vi "数字量输出配置.vi"() -> ()   [LabVIEW 2010] (continued)
              n515 = local write "单选_第67路"(w31) -> ()
              n516 = local write "单选_第68路"(w31) -> ()
              n517 = local write "单选_第69路"(w31) -> ()
              n518 = local write "单选_第70路"(w31) -> ()
              n519 = local write "单选_第72路"(w31) -> ()
              n520 = local write "单选_第73路"(w31) -> ()
              n521 = local write "单选_第74路"(w31) -> ()
              n522 = local write "单选_第75路"(w31) -> ()
              n523 = local write "单选_第76路"(w31) -> ()
              n524 = local write "单选_第77路"(w31) -> ()
              n525 = local write "单选_第78路"(w31) -> ()
              n526 = local write "单选_第80路"(w31) -> ()
            }
            frame 2 {
              w32 = TRUE
              w33 = FALSE ("单选_第41路")
              n527 = local write "单选_第1路"(w32) -> ()
              n528 = local write "单选_第2路"(w32) -> ()
              n529 = local write "单选_第3路"(w33) -> ()
              n530 = local write "单选_第4路"(w33) -> ()
              n531 = local write "单选_第5路"(w33) -> ()
              n532 = local write "单选_第6路"(w33) -> ()
              n533 = local write "单选_第7路"(w33) -> ()
              n534 = local write "单选_第8路"(w33) -> ()
              n535 = local write "单选_第9路"(w33) -> ()
              n536 = local write "单选_第10路"(w33) -> ()
              n537 = local write "单选_第11路"(w33) -> ()
              n538 = local write "单选_第12路"(w33) -> ()
              n539 = local write "单选_第13路"(w33) -> ()
              n540 = local write "单选_第14路"(w33) -> ()
              n541 = local write "单选_第15路"(w33) -> ()
              n542 = local write "单选_第16路"(w33) -> ()
              n543 = local write "单选_第17路"(w33) -> ()
              n544 = local write "单选_第18路"(w33) -> ()
              n545 = local write "单选_第19路"(w33) -> ()
              n546 = local write "单选_第20路"(w33) -> ()
              n547 = local write "单选_第21路"(w33) -> ()
              n548 = local write "单选_第22路"(w33) -> ()
              n549 = local write "单选_第23路"(w33) -> ()
              n550 = local write "单选_第24路"(w33) -> ()
              n551 = local write "单选_第25路"(w33) -> ()
              n552 = local write "单选_第26路"(w33) -> ()
              n553 = local write "单选_第27路"(w33) -> ()
              n554 = local write "单选_第28路"(w33) -> ()
              n555 = local write "单选_第29路"(w33) -> ()
              n556 = local write "单选_第30路"(w33) -> ()
              n557 = local write "单选_第31路"(w33) -> ()
              n558 = local write "单选_第32路"(w33) -> ()
              n559 = local write "单选_第33路"(w33) -> ()
              n560 = local write "单选_第34路"(w33) -> ()
              n561 = local write "单选_第35路"(w33) -> ()
              n562 = local write "单选_第36路"(w33) -> ()
              n563 = local write "单选_第37路"(w33) -> ()
              n564 = local write "单选_第38路"(w33) -> ()
              n565 = local write "单选_第39路"(w33) -> ()
              n566 = local write "单选_第40路"(w33) -> ()
              n567 = local write "单选_第41路"(w33) -> ()
              n568 = local write "单选_第42路"(w33) -> ()
              n569 = local write "单选_第43路"(w33) -> ()
              n570 = local write "单选_第44路"(w33) -> ()
              n571 = local write "单选_第45路"(w33) -> ()
              n572 = local write "单选_第46路"(w33) -> ()
              n573 = local write "单选_第47路"(w33) -> ()
              n574 = local write "单选_第48路"(w33) -> ()
              n575 = local write "单选_第49路"(w33) -> ()
              n576 = local write "单选_第50路"(w33) -> ()
              n577 = local write "单选_第51路"(w33) -> ()
              n578 = local write "单选_第52路"(w33) -> ()
              n579 = local write "单选_第53路"(w33) -> ()
              n580 = local write "单选_第54路"(w33) -> ()
              n581 = local write "单选_第55路"(w33) -> ()
              n582 = local write "单选_第56路"(w33) -> ()
              n583 = local write "单选_第57路"(w33) -> ()
              n584 = local write "单选_第58路"(w33) -> ()
              n585 = local write "单选_第59路"(w33) -> ()
              n586 = local write "单选_第60路"(w33) -> ()
              n587 = local write "单选_第61路"(w33) -> ()
              n588 = local write "单选_第62路"(w33) -> ()
              n589 = local write "单选_第63路"(w33) -> ()
              n590 = local write "单选_第64路"(w33) -> ()
              n591 = local write "单选_第71路"(w33) -> ()
              n592 = local write "单选_第79路"(w33) -> ()
              n593 = local write "单选_第65路"(w33) -> ()
              n594 = local write "单选_第66路"(w33) -> ()
              n595 = local write "单选_第67路"(w33) -> ()
              n596 = local write "单选_第68路"(w33) -> ()
              n597 = local write "单选_第69路"(w33) -> ()
              n598 = local write "单选_第70路"(w33) -> ()
              n599 = local write "单选_第72路"(w33) -> ()
              n600 = local write "单选_第73路"(w33) -> ()
              n601 = local write "单选_第74路"(w33) -> ()
              n602 = local write "单选_第75路"(w33) -> ()
              n603 = local write "单选_第76路"(w33) -> ()
              n604 = local write "单选_第77路"(w33) -> ()
              n605 = local write "单选_第78路"(w33) -> ()
              n606 = local write "单选_第80路"(w33) -> ()
            }
            frame 3 {
              w34 = TRUE
              w35 = FALSE ("单选_第41路")
              n607 = local write "单选_第1路"(w34) -> ()
              n608 = local write "单选_第2路"(w34) -> ()
              n609 = local write "单选_第3路"(w34) -> ()
              n610 = local write "单选_第4路"(w35) -> ()
              n611 = local write "单选_第5路"(w35) -> ()
              n612 = local write "单选_第6路"(w35) -> ()
              n613 = local write "单选_第7路"(w35) -> ()
              n614 = local write "单选_第8路"(w35) -> ()
              n615 = local write "单选_第9路"(w35) -> ()
              n616 = local write "单选_第10路"(w35) -> ()
              n617 = local write "单选_第11路"(w35) -> ()
              n618 = local write "单选_第12路"(w35) -> ()
              n619 = local write "单选_第13路"(w35) -> ()
              n620 = local write "单选_第14路"(w35) -> ()
              n621 = local write "单选_第15路"(w35) -> ()
              n622 = local write "单选_第16路"(w35) -> ()
              n623 = local write "单选_第17路"(w35) -> ()
              n624 = local write "单选_第18路"(w35) -> ()
              n625 = local write "单选_第19路"(w35) -> ()
              n626 = local write "单选_第20路"(w35) -> ()
              n627 = local write "单选_第21路"(w35) -> ()
              n628 = local write "单选_第22路"(w35) -> ()
              n629 = local write "单选_第23路"(w35) -> ()
              n630 = local write "单选_第24路"(w35) -> ()
              n631 = local write "单选_第25路"(w35) -> ()
              n632 = local write "单选_第26路"(w35) -> ()
              n633 = local write "单选_第27路"(w35) -> ()
              n634 = local write "单选_第28路"(w35) -> ()
              n635 = local write "单选_第29路"(w35) -> ()
              n636 = local write "单选_第30路"(w35) -> ()
              n637 = local write "单选_第31路"(w35) -> ()
              n638 = local write "单选_第32路"(w35) -> ()
              n639 = local write "单选_第33路"(w35) -> ()
              n640 = local write "单选_第34路"(w35) -> ()
              n641 = local write "单选_第35路"(w35) -> ()
              n642 = local write "单选_第36路"(w35) -> ()
              n643 = local write "单选_第37路"(w35) -> ()
              n644 = local write "单选_第38路"(w35) -> ()
              n645 = local write "单选_第39路"(w35) -> ()
              n646 = local write "单选_第40路"(w35) -> ()
              n647 = local write "单选_第41路"(w35) -> ()
              n648 = local write "单选_第42路"(w35) -> ()
              n649 = local write "单选_第43路"(w35) -> ()
              n650 = local write "单选_第44路"(w35) -> ()
              n651 = local write "单选_第45路"(w35) -> ()
              n652 = local write "单选_第46路"(w35) -> ()
              n653 = local write "单选_第47路"(w35) -> ()
              n654 = local write "单选_第48路"(w35) -> ()
              n655 = local write "单选_第49路"(w35) -> ()
              n656 = local write "单选_第50路"(w35) -> ()
              n657 = local write "单选_第51路"(w35) -> ()
              n658 = local write "单选_第52路"(w35) -> ()
              n659 = local write "单选_第53路"(w35) -> ()
              n660 = local write "单选_第54路"(w35) -> ()
              n661 = local write "单选_第55路"(w35) -> ()
              n662 = local write "单选_第56路"(w35) -> ()
              n663 = local write "单选_第57路"(w35) -> ()
              n664 = local write "单选_第58路"(w35) -> ()
              n665 = local write "单选_第59路"(w35) -> ()
              n666 = local write "单选_第60路"(w35) -> ()
              n667 = local write "单选_第61路"(w35) -> ()
              n668 = local write "单选_第62路"(w35) -> ()
              n669 = local write "单选_第63路"(w35) -> ()
              n670 = local write "单选_第64路"(w35) -> ()
              n671 = local write "单选_第71路"(w35) -> ()
              n672 = local write "单选_第79路"(w35) -> ()
              n673 = local write "单选_第65路"(w35) -> ()
              n674 = local write "单选_第66路"(w35) -> ()
              n675 = local write "单选_第67路"(w35) -> ()
              n676 = local write "单选_第68路"(w35) -> ()
              n677 = local write "单选_第69路"(w35) -> ()
              n678 = local write "单选_第70路"(w35) -> ()
              n679 = local write "单选_第72路"(w35) -> ()
              n680 = local write "单选_第73路"(w35) -> ()
              n681 = local write "单选_第74路"(w35) -> ()
              n682 = local write "单选_第75路"(w35) -> ()
              n683 = local write "单选_第76路"(w35) -> ()
              n684 = local write "单选_第77路"(w35) -> ()
              n685 = local write "单选_第78路"(w35) -> ()
              n686 = local write "单选_第80路"(w35) -> ()
            }
            frame 4 {
              w36 = TRUE
              w37 = FALSE ("单选_第41路")
              n687 = local write "单选_第1路"(w36) -> ()
              n688 = local write "单选_第2路"(w36) -> ()
              n689 = local write "单选_第3路"(w36) -> ()
              n690 = local write "单选_第4路"(w36) -> ()
              n691 = local write "单选_第5路"(w37) -> ()
              n692 = local write "单选_第6路"(w37) -> ()
              n693 = local write "单选_第7路"(w37) -> ()
              n694 = local write "单选_第8路"(w37) -> ()
              n695 = local write "单选_第9路"(w37) -> ()
              n696 = local write "单选_第10路"(w37) -> ()
              n697 = local write "单选_第11路"(w37) -> ()
              n698 = local write "单选_第12路"(w37) -> ()
              n699 = local write "单选_第13路"(w37) -> ()
              n700 = local write "单选_第14路"(w37) -> ()
              n701 = local write "单选_第15路"(w37) -> ()
              n702 = local write "单选_第16路"(w37) -> ()
              n703 = local write "单选_第17路"(w37) -> ()
              n704 = local write "单选_第18路"(w37) -> ()
              n705 = local write "单选_第19路"(w37) -> ()
              n706 = local write "单选_第20路"(w37) -> ()
              n707 = local write "单选_第21路"(w37) -> ()
              n708 = local write "单选_第22路"(w37) -> ()
              n709 = local write "单选_第23路"(w37) -> ()
              n710 = local write "单选_第24路"(w37) -> ()
              n711 = local write "单选_第25路"(w37) -> ()
              n712 = local write "单选_第26路"(w37) -> ()
              n713 = local write "单选_第27路"(w37) -> ()
              n714 = local write "单选_第28路"(w37) -> ()
              n715 = local write "单选_第29路"(w37) -> ()
              n716 = local write "单选_第30路"(w37) -> ()
              n717 = local write "单选_第31路"(w37) -> ()
              n718 = local write "单选_第32路"(w37) -> ()
              n719 = local write "单选_第33路"(w37) -> ()
              n720 = local write "单选_第34路"(w37) -> ()
              n721 = local write "单选_第35路"(w37) -> ()
              n722 = local write "单选_第36路"(w37) -> ()
              n723 = local write "单选_第37路"(w37) -> ()
              n724 = local write "单选_第38路"(w37) -> ()
              n725 = local write "单选_第39路"(w37) -> ()
              n726 = local write "单选_第40路"(w37) -> ()
              n727 = local write "单选_第41路"(w37) -> ()
              n728 = local write "单选_第42路"(w37) -> ()
              n729 = local write "单选_第43路"(w37) -> ()
              n730 = local write "单选_第44路"(w37) -> ()
              n731 = local write "单选_第45路"(w37) -> ()
              n732 = local write "单选_第46路"(w37) -> ()
              n733 = local write "单选_第47路"(w37) -> ()
              n734 = local write "单选_第48路"(w37) -> ()
              n735 = local write "单选_第49路"(w37) -> ()
              n736 = local write "单选_第50路"(w37) -> ()
              n737 = local write "单选_第51路"(w37) -> ()
              n738 = local write "单选_第52路"(w37) -> ()
              n739 = local write "单选_第53路"(w37) -> ()
              n740 = local write "单选_第54路"(w37) -> ()
              n741 = local write "单选_第55路"(w37) -> ()
              n742 = local write "单选_第56路"(w37) -> ()
              n743 = local write "单选_第57路"(w37) -> ()
              n744 = local write "单选_第58路"(w37) -> ()
              n745 = local write "单选_第59路"(w37) -> ()
              n746 = local write "单选_第60路"(w37) -> ()
              n747 = local write "单选_第61路"(w37) -> ()
              n748 = local write "单选_第62路"(w37) -> ()
              n749 = local write "单选_第63路"(w37) -> ()
              n750 = local write "单选_第64路"(w37) -> ()
              n751 = local write "单选_第71路"(w37) -> ()
              n752 = local write "单选_第79路"(w37) -> ()
              n753 = local write "单选_第65路"(w37) -> ()
              n754 = local write "单选_第66路"(w37) -> ()
              n755 = local write "单选_第67路"(w37) -> ()
              n756 = local write "单选_第68路"(w37) -> ()
              n757 = local write "单选_第69路"(w37) -> ()
              n758 = local write "单选_第70路"(w37) -> ()
              n759 = local write "单选_第72路"(w37) -> ()
              n760 = local write "单选_第73路"(w37) -> ()
              n761 = local write "单选_第74路"(w37) -> ()
              n762 = local write "单选_第75路"(w37) -> ()
              n763 = local write "单选_第76路"(w37) -> ()
              n764 = local write "单选_第77路"(w37) -> ()
              n765 = local write "单选_第78路"(w37) -> ()
              n766 = local write "单选_第80路"(w37) -> ()
            }
            frame 5 {
              w38 = TRUE
              w39 = FALSE ("单选_第41路")
              n767 = local write "单选_第1路"(w38) -> ()
              n768 = local write "单选_第2路"(w38) -> ()
              n769 = local write "单选_第3路"(w38) -> ()
              n770 = local write "单选_第4路"(w38) -> ()
              n771 = local write "单选_第5路"(w38) -> ()
              n772 = local write "单选_第6路"(w39) -> ()
              n773 = local write "单选_第7路"(w39) -> ()
              n774 = local write "单选_第8路"(w39) -> ()
              n775 = local write "单选_第9路"(w39) -> ()
              n776 = local write "单选_第10路"(w39) -> ()
              n777 = local write "单选_第11路"(w39) -> ()
              n778 = local write "单选_第12路"(w39) -> ()
              n779 = local write "单选_第13路"(w39) -> ()
              n780 = local write "单选_第14路"(w39) -> ()
              n781 = local write "单选_第15路"(w39) -> ()
              n782 = local write "单选_第16路"(w39) -> ()
              n783 = local write "单选_第17路"(w39) -> ()
              n784 = local write "单选_第18路"(w39) -> ()
              n785 = local write "单选_第19路"(w39) -> ()
              n786 = local write "单选_第20路"(w39) -> ()
              n787 = local write "单选_第21路"(w39) -> ()
              n788 = local write "单选_第22路"(w39) -> ()
              n789 = local write "单选_第23路"(w39) -> ()
              n790 = local write "单选_第24路"(w39) -> ()
              n791 = local write "单选_第25路"(w39) -> ()
              n792 = local write "单选_第26路"(w39) -> ()
              n793 = local write "单选_第27路"(w39) -> ()
              n794 = local write "单选_第28路"(w39) -> ()
              n795 = local write "单选_第29路"(w39) -> ()
              n796 = local write "单选_第30路"(w39) -> ()
              n797 = local write "单选_第31路"(w39) -> ()
              n798 = local write "单选_第32路"(w39) -> ()
              n799 = local write "单选_第33路"(w39) -> ()
              n800 = local write "单选_第34路"(w39) -> ()
              n801 = local write "单选_第35路"(w39) -> ()
              n802 = local write "单选_第36路"(w39) -> ()
              n803 = local write "单选_第37路"(w39) -> ()
              n804 = local write "单选_第38路"(w39) -> ()
              n805 = local write "单选_第39路"(w39) -> ()
              n806 = local write "单选_第40路"(w39) -> ()
              n807 = local write "单选_第41路"(w39) -> ()
              n808 = local write "单选_第42路"(w39) -> ()
              n809 = local write "单选_第43路"(w39) -> ()
              n810 = local write "单选_第44路"(w39) -> ()
              n811 = local write "单选_第45路"(w39) -> ()
              n812 = local write "单选_第46路"(w39) -> ()
              n813 = local write "单选_第47路"(w39) -> ()
              n814 = local write "单选_第48路"(w39) -> ()
              n815 = local write "单选_第49路"(w39) -> ()
              n816 = local write "单选_第50路"(w39) -> ()
              n817 = local write "单选_第51路"(w39) -> ()
              n818 = local write "单选_第52路"(w39) -> ()
              n819 = local write "单选_第53路"(w39) -> ()
              n820 = local write "单选_第54路"(w39) -> ()
              n821 = local write "单选_第55路"(w39) -> ()
              n822 = local write "单选_第56路"(w39) -> ()
              n823 = local write "单选_第57路"(w39) -> ()
              n824 = local write "单选_第58路"(w39) -> ()
              n825 = local write "单选_第59路"(w39) -> ()
              n826 = local write "单选_第60路"(w39) -> ()
              n827 = local write "单选_第61路"(w39) -> ()
              n828 = local write "单选_第62路"(w39) -> ()
              n829 = local write "单选_第63路"(w39) -> ()
              n830 = local write "单选_第64路"(w39) -> ()
              n831 = local write "单选_第71路"(w39) -> ()
              n832 = local write "单选_第79路"(w39) -> ()
              n833 = local write "单选_第65路"(w39) -> ()
              n834 = local write "单选_第66路"(w39) -> ()
              n835 = local write "单选_第67路"(w39) -> ()
              n836 = local write "单选_第68路"(w39) -> ()
              n837 = local write "单选_第69路"(w39) -> ()
              n838 = local write "单选_第70路"(w39) -> ()
              n839 = local write "单选_第72路"(w39) -> ()
              n840 = local write "单选_第73路"(w39) -> ()
              n841 = local write "单选_第74路"(w39) -> ()
              n842 = local write "单选_第75路"(w39) -> ()
              n843 = local write "单选_第76路"(w39) -> ()
              n844 = local write "单选_第77路"(w39) -> ()
              n845 = local write "单选_第78路"(w39) -> ()
              n846 = local write "单选_第80路"(w39) -> ()
            }
            frame 6 {
              w40 = TRUE
              w41 = FALSE ("单选_第41路")
              n847 = local write "单选_第1路"(w40) -> ()
              n848 = local write "单选_第2路"(w40) -> ()
              n849 = local write "单选_第3路"(w40) -> ()
              n850 = local write "单选_第4路"(w40) -> ()
              n851 = local write "单选_第5路"(w40) -> ()
              n852 = local write "单选_第6路"(w40) -> ()
              n853 = local write "单选_第7路"(w41) -> ()
              n854 = local write "单选_第8路"(w41) -> ()
              n855 = local write "单选_第9路"(w41) -> ()
              n856 = local write "单选_第10路"(w41) -> ()
              n857 = local write "单选_第11路"(w41) -> ()
              n858 = local write "单选_第12路"(w41) -> ()
              n859 = local write "单选_第13路"(w41) -> ()
              n860 = local write "单选_第14路"(w41) -> ()
              n861 = local write "单选_第15路"(w41) -> ()
              n862 = local write "单选_第16路"(w41) -> ()
              n863 = local write "单选_第17路"(w41) -> ()
              n864 = local write "单选_第18路"(w41) -> ()
              n865 = local write "单选_第19路"(w41) -> ()
              n866 = local write "单选_第20路"(w41) -> ()
              n867 = local write "单选_第21路"(w41) -> ()
              n868 = local write "单选_第22路"(w41) -> ()
              n869 = local write "单选_第23路"(w41) -> ()
              n870 = local write "单选_第24路"(w41) -> ()
              n871 = local write "单选_第25路"(w41) -> ()
              n872 = local write "单选_第26路"(w41) -> ()
              n873 = local write "单选_第27路"(w41) -> ()
              n874 = local write "单选_第28路"(w41) -> ()
              n875 = local write "单选_第29路"(w41) -> ()
              n876 = local write "单选_第30路"(w41) -> ()
              n877 = local write "单选_第31路"(w41) -> ()
              n878 = local write "单选_第32路"(w41) -> ()
              n879 = local write "单选_第33路"(w41) -> ()
              n880 = local write "单选_第34路"(w41) -> ()
              n881 = local write "单选_第35路"(w41) -> ()
              n882 = local write "单选_第36路"(w41) -> ()
              n883 = local write "单选_第37路"(w41) -> ()
              n884 = local write "单选_第38路"(w41) -> ()
              n885 = local write "单选_第39路"(w41) -> ()
              n886 = local write "单选_第40路"(w41) -> ()
              n887 = local write "单选_第41路"(w41) -> ()
              n888 = local write "单选_第42路"(w41) -> ()
              n889 = local write "单选_第43路"(w41) -> ()
              n890 = local write "单选_第44路"(w41) -> ()
              n891 = local write "单选_第45路"(w41) -> ()
              n892 = local write "单选_第46路"(w41) -> ()
              n893 = local write "单选_第47路"(w41) -> ()
              n894 = local write "单选_第48路"(w41) -> ()
              n895 = local write "单选_第49路"(w41) -> ()
              n896 = local write "单选_第50路"(w41) -> ()
              n897 = local write "单选_第51路"(w41) -> ()
              n898 = local write "单选_第52路"(w41) -> ()
              n899 = local write "单选_第53路"(w41) -> ()
              n900 = local write "单选_第54路"(w41) -> ()
              n901 = local write "单选_第55路"(w41) -> ()
              n902 = local write "单选_第56路"(w41) -> ()
              n903 = local write "单选_第57路"(w41) -> ()
              n904 = local write "单选_第58路"(w41) -> ()
              n905 = local write "单选_第59路"(w41) -> ()
              n906 = local write "单选_第60路"(w41) -> ()
              n907 = local write "单选_第61路"(w41) -> ()
              n908 = local write "单选_第62路"(w41) -> ()
              n909 = local write "单选_第63路"(w41) -> ()
              n910 = local write "单选_第64路"(w41) -> ()
              n911 = local write "单选_第71路"(w41) -> ()
              n912 = local write "单选_第79路"(w41) -> ()
              n913 = local write "单选_第65路"(w41) -> ()
              n914 = local write "单选_第66路"(w41) -> ()
              n915 = local write "单选_第67路"(w41) -> ()
              n916 = local write "单选_第68路"(w41) -> ()
              n917 = local write "单选_第69路"(w41) -> ()
              n918 = local write "单选_第70路"(w41) -> ()
              n919 = local write "单选_第72路"(w41) -> ()
              n920 = local write "单选_第73路"(w41) -> ()
              n921 = local write "单选_第74路"(w41) -> ()
              n922 = local write "单选_第75路"(w41) -> ()
              n923 = local write "单选_第76路"(w41) -> ()
              n924 = local write "单选_第77路"(w41) -> ()
              n925 = local write "单选_第78路"(w41) -> ()
              n926 = local write "单选_第80路"(w41) -> ()
            }
            frame 7 {
              w42 = TRUE
              w43 = FALSE ("单选_第41路")
              n927 = local write "单选_第1路"(w42) -> ()
              n928 = local write "单选_第2路"(w42) -> ()
              n929 = local write "单选_第3路"(w42) -> ()
              n930 = local write "单选_第4路"(w42) -> ()
              n931 = local write "单选_第5路"(w42) -> ()
              n932 = local write "单选_第6路"(w42) -> ()
              n933 = local write "单选_第7路"(w42) -> ()
              n934 = local write "单选_第8路"(w43) -> ()
              n935 = local write "单选_第9路"(w43) -> ()
              n936 = local write "单选_第10路"(w43) -> ()
              n937 = local write "单选_第11路"(w43) -> ()
              n938 = local write "单选_第12路"(w43) -> ()
              n939 = local write "单选_第13路"(w43) -> ()
              n940 = local write "单选_第14路"(w43) -> ()
              n941 = local write "单选_第15路"(w43) -> ()
              n942 = local write "单选_第16路"(w43) -> ()
              n943 = local write "单选_第17路"(w43) -> ()
              n944 = local write "单选_第18路"(w43) -> ()
              n945 = local write "单选_第19路"(w43) -> ()
              n946 = local write "单选_第20路"(w43) -> ()
              n947 = local write "单选_第21路"(w43) -> ()
              n948 = local write "单选_第22路"(w43) -> ()
              n949 = local write "单选_第23路"(w43) -> ()
              n950 = local write "单选_第24路"(w43) -> ()
              n951 = local write "单选_第25路"(w43) -> ()
              n952 = local write "单选_第26路"(w43) -> ()
              n953 = local write "单选_第27路"(w43) -> ()
              n954 = local write "单选_第28路"(w43) -> ()
              n955 = local write "单选_第29路"(w43) -> ()
              n956 = local write "单选_第30路"(w43) -> ()
              n957 = local write "单选_第31路"(w43) -> ()
              n958 = local write "单选_第32路"(w43) -> ()
              n959 = local write "单选_第33路"(w43) -> ()
              n960 = local write "单选_第34路"(w43) -> ()
              n961 = local write "单选_第35路"(w43) -> ()
              n962 = local write "单选_第36路"(w43) -> ()
              n963 = local write "单选_第37路"(w43) -> ()
              n964 = local write "单选_第38路"(w43) -> ()
              n965 = local write "单选_第39路"(w43) -> ()
              n966 = local write "单选_第40路"(w43) -> ()
              n967 = local write "单选_第41路"(w43) -> ()
              n968 = local write "单选_第42路"(w43) -> ()
              n969 = local write "单选_第43路"(w43) -> ()
              n970 = local write "单选_第44路"(w43) -> ()
              n971 = local write "单选_第45路"(w43) -> ()
              n972 = local write "单选_第46路"(w43) -> ()
              n973 = local write "单选_第47路"(w43) -> ()
              n974 = local write "单选_第48路"(w43) -> ()
              n975 = local write "单选_第49路"(w43) -> ()
              n976 = local write "单选_第50路"(w43) -> ()
              n977 = local write "单选_第51路"(w43) -> ()
              n978 = local write "单选_第52路"(w43) -> ()
              n979 = local write "单选_第53路"(w43) -> ()
              n980 = local write "单选_第54路"(w43) -> ()
              n981 = local write "单选_第55路"(w43) -> ()
              n982 = local write "单选_第56路"(w43) -> ()
              n983 = local write "单选_第57路"(w43) -> ()
              n984 = local write "单选_第58路"(w43) -> ()
              n985 = local write "单选_第59路"(w43) -> ()
              n986 = local write "单选_第60路"(w43) -> ()
              n987 = local write "单选_第61路"(w43) -> ()
              n988 = local write "单选_第62路"(w43) -> ()
              n989 = local write "单选_第63路"(w43) -> ()
              n990 = local write "单选_第64路"(w43) -> ()
              n991 = local write "单选_第71路"(w43) -> ()
              n992 = local write "单选_第79路"(w43) -> ()
              n993 = local write "单选_第65路"(w43) -> ()
              n994 = local write "单选_第66路"(w43) -> ()
              n995 = local write "单选_第67路"(w43) -> ()
              n996 = local write "单选_第68路"(w43) -> ()
              n997 = local write "单选_第69路"(w43) -> ()
              n998 = local write "单选_第70路"(w43) -> ()
              n999 = local write "单选_第72路"(w43) -> ()
              n1000 = local write "单选_第73路"(w43) -> ()
              n1001 = local write "单选_第74路"(w43) -> ()
              n1002 = local write "单选_第75路"(w43) -> ()
              n1003 = local write "单选_第76路"(w43) -> ()
              n1004 = local write "单选_第77路"(w43) -> ()
              n1005 = local write "单选_第78路"(w43) -> ()
              n1006 = local write "单选_第80路"(w43) -> ()
            }
            frame 8 {
              w44 = TRUE
              w45 = FALSE ("单选_第41路")
              n1007 = local write "单选_第1路"(w44) -> ()
              n1008 = local write "单选_第2路"(w44) -> ()
              n1009 = local write "单选_第3路"(w44) -> ()
              n1010 = local write "单选_第4路"(w44) -> ()
              n1011 = local write "单选_第5路"(w44) -> ()
              n1012 = local write "单选_第6路"(w44) -> ()
              n1013 = local write "单选_第7路"(w44) -> ()
              n1014 = local write "单选_第8路"(w44) -> ()
              n1015 = local write "单选_第9路"(w45) -> ()
              n1016 = local write "单选_第10路"(w45) -> ()
              n1017 = local write "单选_第11路"(w45) -> ()
              n1018 = local write "单选_第12路"(w45) -> ()
              n1019 = local write "单选_第13路"(w45) -> ()
              n1020 = local write "单选_第14路"(w45) -> ()
              n1021 = local write "单选_第15路"(w45) -> ()
              n1022 = local write "单选_第16路"(w45) -> ()
              n1023 = local write "单选_第17路"(w45) -> ()
              n1024 = local write "单选_第18路"(w45) -> ()
              n1025 = local write "单选_第19路"(w45) -> ()
              n1026 = local write "单选_第20路"(w45) -> ()
              n1027 = local write "单选_第21路"(w45) -> ()
              n1028 = local write "单选_第22路"(w45) -> ()
              n1029 = local write "单选_第23路"(w45) -> ()
              n1030 = local write "单选_第24路"(w45) -> ()
              n1031 = local write "单选_第25路"(w45) -> ()
              n1032 = local write "单选_第26路"(w45) -> ()
              n1033 = local write "单选_第27路"(w45) -> ()
              n1034 = local write "单选_第28路"(w45) -> ()
              n1035 = local write "单选_第29路"(w45) -> ()
              n1036 = local write "单选_第30路"(w45) -> ()
              n1037 = local write "单选_第31路"(w45) -> ()
              n1038 = local write "单选_第32路"(w45) -> ()
              n1039 = local write "单选_第33路"(w45) -> ()
              n1040 = local write "单选_第34路"(w45) -> ()
              n1041 = local write "单选_第35路"(w45) -> ()
              n1042 = local write "单选_第36路"(w45) -> ()
              n1043 = local write "单选_第37路"(w45) -> ()
              n1044 = local write "单选_第38路"(w45) -> ()
              n1045 = local write "单选_第39路"(w45) -> ()
              n1046 = local write "单选_第40路"(w45) -> ()
              n1047 = local write "单选_第41路"(w45) -> ()
              n1048 = local write "单选_第42路"(w45) -> ()
              n1049 = local write "单选_第43路"(w45) -> ()
              n1050 = local write "单选_第44路"(w45) -> ()
              n1051 = local write "单选_第45路"(w45) -> ()
              n1052 = local write "单选_第46路"(w45) -> ()
              n1053 = local write "单选_第47路"(w45) -> ()
              n1054 = local write "单选_第48路"(w45) -> ()
              n1055 = local write "单选_第49路"(w45) -> ()
              n1056 = local write "单选_第50路"(w45) -> ()
              n1057 = local write "单选_第51路"(w45) -> ()
              n1058 = local write "单选_第52路"(w45) -> ()
              n1059 = local write "单选_第53路"(w45) -> ()
              n1060 = local write "单选_第54路"(w45) -> ()
              n1061 = local write "单选_第55路"(w45) -> ()
              n1062 = local write "单选_第56路"(w45) -> ()
              n1063 = local write "单选_第57路"(w45) -> ()
              n1064 = local write "单选_第58路"(w45) -> ()
              n1065 = local write "单选_第59路"(w45) -> ()
              n1066 = local write "单选_第60路"(w45) -> ()
              n1067 = local write "单选_第61路"(w45) -> ()
              n1068 = local write "单选_第62路"(w45) -> ()
              n1069 = local write "单选_第63路"(w45) -> ()
              n1070 = local write "单选_第64路"(w45) -> ()
              n1071 = local write "单选_第71路"(w45) -> ()
              n1072 = local write "单选_第79路"(w45) -> ()
              n1073 = local write "单选_第65路"(w45) -> ()
              n1074 = local write "单选_第66路"(w45) -> ()
              n1075 = local write "单选_第67路"(w45) -> ()
              n1076 = local write "单选_第68路"(w45) -> ()
              n1077 = local write "单选_第69路"(w45) -> ()
              n1078 = local write "单选_第70路"(w45) -> ()
              n1079 = local write "单选_第72路"(w45) -> ()
              n1080 = local write "单选_第73路"(w45) -> ()
              n1081 = local write "单选_第74路"(w45) -> ()
              n1082 = local write "单选_第75路"(w45) -> ()
              n1083 = local write "单选_第76路"(w45) -> ()
              n1084 = local write "单选_第77路"(w45) -> ()
              n1085 = local write "单选_第78路"(w45) -> ()
              n1086 = local write "单选_第80路"(w45) -> ()
            }
            frame 9 {
              w46 = TRUE
              w47 = FALSE ("单选_第41路")
              n1087 = local write "单选_第1路"(w46) -> ()
              n1088 = local write "单选_第2路"(w46) -> ()
              n1089 = local write "单选_第3路"(w46) -> ()
              n1090 = local write "单选_第4路"(w46) -> ()
              n1091 = local write "单选_第5路"(w46) -> ()
              n1092 = local write "单选_第6路"(w46) -> ()
              n1093 = local write "单选_第7路"(w46) -> ()
              n1094 = local write "单选_第8路"(w46) -> ()
              n1095 = local write "单选_第9路"(w46) -> ()
              n1096 = local write "单选_第10路"(w47) -> ()
              n1097 = local write "单选_第11路"(w47) -> ()
              n1098 = local write "单选_第12路"(w47) -> ()
              n1099 = local write "单选_第13路"(w47) -> ()
              n1100 = local write "单选_第14路"(w47) -> ()
              n1101 = local write "单选_第15路"(w47) -> ()
              n1102 = local write "单选_第16路"(w47) -> ()
              n1103 = local write "单选_第17路"(w47) -> ()
              n1104 = local write "单选_第18路"(w47) -> ()
              n1105 = local write "单选_第19路"(w47) -> ()
              n1106 = local write "单选_第20路"(w47) -> ()
              n1107 = local write "单选_第21路"(w47) -> ()
              n1108 = local write "单选_第22路"(w47) -> ()
              n1109 = local write "单选_第23路"(w47) -> ()
              n1110 = local write "单选_第24路"(w47) -> ()
              n1111 = local write "单选_第25路"(w47) -> ()
              n1112 = local write "单选_第26路"(w47) -> ()
              n1113 = local write "单选_第27路"(w47) -> ()
              n1114 = local write "单选_第28路"(w47) -> ()
              n1115 = local write "单选_第29路"(w47) -> ()
              n1116 = local write "单选_第30路"(w47) -> ()
              n1117 = local write "单选_第31路"(w47) -> ()
              n1118 = local write "单选_第32路"(w47) -> ()
              n1119 = local write "单选_第33路"(w47) -> ()
              n1120 = local write "单选_第34路"(w47) -> ()
              n1121 = local write "单选_第35路"(w47) -> ()
              n1122 = local write "单选_第36路"(w47) -> ()
              n1123 = local write "单选_第37路"(w47) -> ()
              n1124 = local write "单选_第38路"(w47) -> ()
              n1125 = local write "单选_第39路"(w47) -> ()
              n1126 = local write "单选_第40路"(w47) -> ()
              n1127 = local write "单选_第41路"(w47) -> ()
              n1128 = local write "单选_第42路"(w47) -> ()
              n1129 = local write "单选_第43路"(w47) -> ()
              n1130 = local write "单选_第44路"(w47) -> ()
              n1131 = local write "单选_第45路"(w47) -> ()
              n1132 = local write "单选_第46路"(w47) -> ()
              n1133 = local write "单选_第47路"(w47) -> ()
              n1134 = local write "单选_第48路"(w47) -> ()
              n1135 = local write "单选_第49路"(w47) -> ()
              n1136 = local write "单选_第50路"(w47) -> ()
              n1137 = local write "单选_第51路"(w47) -> ()
              n1138 = local write "单选_第52路"(w47) -> ()
              n1139 = local write "单选_第53路"(w47) -> ()
              n1140 = local write "单选_第54路"(w47) -> ()
              n1141 = local write "单选_第55路"(w47) -> ()
              n1142 = local write "单选_第56路"(w47) -> ()
              n1143 = local write "单选_第57路"(w47) -> ()
              n1144 = local write "单选_第58路"(w47) -> ()
              n1145 = local write "单选_第59路"(w47) -> ()
              n1146 = local write "单选_第60路"(w47) -> ()
              n1147 = local write "单选_第61路"(w47) -> ()
              n1148 = local write "单选_第62路"(w47) -> ()
              n1149 = local write "单选_第63路"(w47) -> ()
              n1150 = local write "单选_第64路"(w47) -> ()
              n1151 = local write "单选_第71路"(w47) -> ()
              n1152 = local write "单选_第79路"(w47) -> ()
              n1153 = local write "单选_第65路"(w47) -> ()
              n1154 = local write "单选_第66路"(w47) -> ()
              n1155 = local write "单选_第67路"(w47) -> ()
              n1156 = local write "单选_第68路"(w47) -> ()
              n1157 = local write "单选_第69路"(w47) -> ()
              n1158 = local write "单选_第70路"(w47) -> ()
              n1159 = local write "单选_第72路"(w47) -> ()
              n1160 = local write "单选_第73路"(w47) -> ()
              n1161 = local write "单选_第74路"(w47) -> ()
              n1162 = local write "单选_第75路"(w47) -> ()
              n1163 = local write "单选_第76路"(w47) -> ()
              n1164 = local write "单选_第77路"(w47) -> ()
              n1165 = local write "单选_第78路"(w47) -> ()
              n1166 = local write "单选_第80路"(w47) -> ()
            }
            frame 10 {
              w48 = TRUE
              w49 = FALSE ("单选_第41路")
              n1167 = local write "单选_第1路"(w48) -> ()
              n1168 = local write "单选_第2路"(w48) -> ()
              n1169 = local write "单选_第3路"(w48) -> ()
              n1170 = local write "单选_第4路"(w48) -> ()
              n1171 = local write "单选_第5路"(w48) -> ()
              n1172 = local write "单选_第6路"(w48) -> ()
              n1173 = local write "单选_第7路"(w48) -> ()
              n1174 = local write "单选_第8路"(w48) -> ()
              n1175 = local write "单选_第9路"(w48) -> ()
              n1176 = local write "单选_第10路"(w48) -> ()
              n1177 = local write "单选_第11路"(w49) -> ()
              n1178 = local write "单选_第12路"(w49) -> ()
              n1179 = local write "单选_第13路"(w49) -> ()
              n1180 = local write "单选_第14路"(w49) -> ()
              n1181 = local write "单选_第15路"(w49) -> ()
              n1182 = local write "单选_第16路"(w49) -> ()
              n1183 = local write "单选_第17路"(w49) -> ()
              n1184 = local write "单选_第18路"(w49) -> ()
              n1185 = local write "单选_第19路"(w49) -> ()
              n1186 = local write "单选_第20路"(w49) -> ()
              n1187 = local write "单选_第21路"(w49) -> ()
              n1188 = local write "单选_第22路"(w49) -> ()
              n1189 = local write "单选_第23路"(w49) -> ()
              n1190 = local write "单选_第24路"(w49) -> ()
              n1191 = local write "单选_第25路"(w49) -> ()
              n1192 = local write "单选_第26路"(w49) -> ()
              n1193 = local write "单选_第27路"(w49) -> ()
              n1194 = local write "单选_第28路"(w49) -> ()
              n1195 = local write "单选_第29路"(w49) -> ()
              n1196 = local write "单选_第30路"(w49) -> ()
              n1197 = local write "单选_第31路"(w49) -> ()
              n1198 = local write "单选_第32路"(w49) -> ()
              n1199 = local write "单选_第33路"(w49) -> ()
              n1200 = local write "单选_第34路"(w49) -> ()
              n1201 = local write "单选_第35路"(w49) -> ()
              n1202 = local write "单选_第36路"(w49) -> ()
              n1203 = local write "单选_第37路"(w49) -> ()
              n1204 = local write "单选_第38路"(w49) -> ()
              n1205 = local write "单选_第39路"(w49) -> ()
              n1206 = local write "单选_第40路"(w49) -> ()
              n1207 = local write "单选_第41路"(w49) -> ()
              n1208 = local write "单选_第42路"(w49) -> ()
              n1209 = local write "单选_第43路"(w49) -> ()
              n1210 = local write "单选_第44路"(w49) -> ()
              n1211 = local write "单选_第45路"(w49) -> ()
              n1212 = local write "单选_第46路"(w49) -> ()
              n1213 = local write "单选_第47路"(w49) -> ()
              n1214 = local write "单选_第48路"(w49) -> ()
              n1215 = local write "单选_第49路"(w49) -> ()
              n1216 = local write "单选_第50路"(w49) -> ()
              n1217 = local write "单选_第51路"(w49) -> ()
              n1218 = local write "单选_第52路"(w49) -> ()
              n1219 = local write "单选_第53路"(w49) -> ()
              n1220 = local write "单选_第54路"(w49) -> ()
              n1221 = local write "单选_第55路"(w49) -> ()
              n1222 = local write "单选_第56路"(w49) -> ()
              n1223 = local write "单选_第57路"(w49) -> ()
              n1224 = local write "单选_第58路"(w49) -> ()
              n1225 = local write "单选_第59路"(w49) -> ()
              n1226 = local write "单选_第60路"(w49) -> ()
              n1227 = local write "单选_第61路"(w49) -> ()
              n1228 = local write "单选_第62路"(w49) -> ()
              n1229 = local write "单选_第63路"(w49) -> ()
              n1230 = local write "单选_第64路"(w49) -> ()
              n1231 = local write "单选_第71路"(w49) -> ()
              n1232 = local write "单选_第79路"(w49) -> ()
              n1233 = local write "单选_第65路"(w49) -> ()
              n1234 = local write "单选_第66路"(w49) -> ()
              n1235 = local write "单选_第67路"(w49) -> ()
              n1236 = local write "单选_第68路"(w49) -> ()
              n1237 = local write "单选_第69路"(w49) -> ()
              n1238 = local write "单选_第70路"(w49) -> ()
              n1239 = local write "单选_第72路"(w49) -> ()
              n1240 = local write "单选_第73路"(w49) -> ()
              n1241 = local write "单选_第74路"(w49) -> ()
              n1242 = local write "单选_第75路"(w49) -> ()
              n1243 = local write "单选_第76路"(w49) -> ()
              n1244 = local write "单选_第77路"(w49) -> ()
              n1245 = local write "单选_第78路"(w49) -> ()
              n1246 = local write "单选_第80路"(w49) -> ()
            }
            frame 11 {
              w50 = TRUE
              w51 = FALSE ("单选_第41路")
              n1247 = local write "单选_第1路"(w50) -> ()
              n1248 = local write "单选_第2路"(w50) -> ()
              n1249 = local write "单选_第3路"(w50) -> ()
              n1250 = local write "单选_第4路"(w50) -> ()
              n1251 = local write "单选_第5路"(w50) -> ()
              n1252 = local write "单选_第6路"(w50) -> ()
              n1253 = local write "单选_第7路"(w50) -> ()
              n1254 = local write "单选_第8路"(w50) -> ()
              n1255 = local write "单选_第9路"(w50) -> ()
              n1256 = local write "单选_第10路"(w50) -> ()
              n1257 = local write "单选_第11路"(w50) -> ()
              n1258 = local write "单选_第12路"(w51) -> ()
              n1259 = local write "单选_第13路"(w51) -> ()
              n1260 = local write "单选_第14路"(w51) -> ()
              n1261 = local write "单选_第15路"(w51) -> ()
              n1262 = local write "单选_第16路"(w51) -> ()
              n1263 = local write "单选_第17路"(w51) -> ()
              n1264 = local write "单选_第18路"(w51) -> ()
              n1265 = local write "单选_第19路"(w51) -> ()
              n1266 = local write "单选_第20路"(w51) -> ()
              n1267 = local write "单选_第21路"(w51) -> ()
              n1268 = local write "单选_第22路"(w51) -> ()
              n1269 = local write "单选_第23路"(w51) -> ()
              n1270 = local write "单选_第24路"(w51) -> ()
              n1271 = local write "单选_第25路"(w51) -> ()
              n1272 = local write "单选_第26路"(w51) -> ()
              n1273 = local write "单选_第27路"(w51) -> ()
              n1274 = local write "单选_第28路"(w51) -> ()
              n1275 = local write "单选_第29路"(w51) -> ()
              n1276 = local write "单选_第30路"(w51) -> ()
              n1277 = local write "单选_第31路"(w51) -> ()
              n1278 = local write "单选_第32路"(w51) -> ()
              n1279 = local write "单选_第33路"(w51) -> ()
              n1280 = local write "单选_第34路"(w51) -> ()
              n1281 = local write "单选_第35路"(w51) -> ()
              n1282 = local write "单选_第36路"(w51) -> ()
              n1283 = local write "单选_第37路"(w51) -> ()
              n1284 = local write "单选_第38路"(w51) -> ()
              n1285 = local write "单选_第39路"(w51) -> ()
              n1286 = local write "单选_第40路"(w51) -> ()
              n1287 = local write "单选_第41路"(w51) -> ()
              n1288 = local write "单选_第42路"(w51) -> ()
              n1289 = local write "单选_第43路"(w51) -> ()
              n1290 = local write "单选_第44路"(w51) -> ()
              n1291 = local write "单选_第45路"(w51) -> ()
              n1292 = local write "单选_第46路"(w51) -> ()
              n1293 = local write "单选_第47路"(w51) -> ()
              n1294 = local write "单选_第48路"(w51) -> ()
              n1295 = local write "单选_第49路"(w51) -> ()
              n1296 = local write "单选_第50路"(w51) -> ()
              n1297 = local write "单选_第51路"(w51) -> ()
              n1298 = local write "单选_第52路"(w51) -> ()
              n1299 = local write "单选_第53路"(w51) -> ()
              n1300 = local write "单选_第54路"(w51) -> ()
              n1301 = local write "单选_第55路"(w51) -> ()
              n1302 = local write "单选_第56路"(w51) -> ()
              n1303 = local write "单选_第57路"(w51) -> ()
              n1304 = local write "单选_第58路"(w51) -> ()
              n1305 = local write "单选_第59路"(w51) -> ()
              n1306 = local write "单选_第60路"(w51) -> ()
              n1307 = local write "单选_第61路"(w51) -> ()
              n1308 = local write "单选_第62路"(w51) -> ()
              n1309 = local write "单选_第63路"(w51) -> ()
              n1310 = local write "单选_第64路"(w51) -> ()
              n1311 = local write "单选_第71路"(w51) -> ()
              n1312 = local write "单选_第79路"(w51) -> ()
              n1313 = local write "单选_第65路"(w51) -> ()
              n1314 = local write "单选_第66路"(w51) -> ()
              n1315 = local write "单选_第67路"(w51) -> ()
              n1316 = local write "单选_第68路"(w51) -> ()
              n1317 = local write "单选_第69路"(w51) -> ()
              n1318 = local write "单选_第70路"(w51) -> ()
              n1319 = local write "单选_第72路"(w51) -> ()
              n1320 = local write "单选_第73路"(w51) -> ()
              n1321 = local write "单选_第74路"(w51) -> ()
              n1322 = local write "单选_第75路"(w51) -> ()
              n1323 = local write "单选_第76路"(w51) -> ()
              n1324 = local write "单选_第77路"(w51) -> ()
              n1325 = local write "单选_第78路"(w51) -> ()
              n1326 = local write "单选_第80路"(w51) -> ()
            }
            frame 12 {
              w52 = TRUE
              w53 = FALSE ("单选_第41路")
              n1327 = local write "单选_第1路"(w52) -> ()
              n1328 = local write "单选_第2路"(w52) -> ()
              n1329 = local write "单选_第3路"(w52) -> ()
              n1330 = local write "单选_第4路"(w52) -> ()
              n1331 = local write "单选_第5路"(w52) -> ()
              n1332 = local write "单选_第6路"(w52) -> ()
              n1333 = local write "单选_第7路"(w52) -> ()
              n1334 = local write "单选_第8路"(w52) -> ()
              n1335 = local write "单选_第9路"(w52) -> ()
              n1336 = local write "单选_第10路"(w52) -> ()
              n1337 = local write "单选_第11路"(w52) -> ()
              n1338 = local write "单选_第12路"(w52) -> ()
              n1339 = local write "单选_第13路"(w53) -> ()
              n1340 = local write "单选_第14路"(w53) -> ()
              n1341 = local write "单选_第15路"(w53) -> ()
              n1342 = local write "单选_第16路"(w53) -> ()
              n1343 = local write "单选_第17路"(w53) -> ()
              n1344 = local write "单选_第18路"(w53) -> ()
              n1345 = local write "单选_第19路"(w53) -> ()
              n1346 = local write "单选_第20路"(w53) -> ()
              n1347 = local write "单选_第21路"(w53) -> ()
              n1348 = local write "单选_第22路"(w53) -> ()
              n1349 = local write "单选_第23路"(w53) -> ()
              n1350 = local write "单选_第24路"(w53) -> ()
              n1351 = local write "单选_第25路"(w53) -> ()
              n1352 = local write "单选_第26路"(w53) -> ()
              n1353 = local write "单选_第27路"(w53) -> ()
              n1354 = local write "单选_第28路"(w53) -> ()
              n1355 = local write "单选_第29路"(w53) -> ()
              n1356 = local write "单选_第30路"(w53) -> ()
              n1357 = local write "单选_第31路"(w53) -> ()
              n1358 = local write "单选_第32路"(w53) -> ()
              n1359 = local write "单选_第33路"(w53) -> ()
              n1360 = local write "单选_第34路"(w53) -> ()
              n1361 = local write "单选_第35路"(w53) -> ()
              n1362 = local write "单选_第36路"(w53) -> ()
              n1363 = local write "单选_第37路"(w53) -> ()
              n1364 = local write "单选_第38路"(w53) -> ()
              n1365 = local write "单选_第39路"(w53) -> ()
              n1366 = local write "单选_第40路"(w53) -> ()
              n1367 = local write "单选_第41路"(w53) -> ()
              n1368 = local write "单选_第42路"(w53) -> ()
              n1369 = local write "单选_第43路"(w53) -> ()
              n1370 = local write "单选_第44路"(w53) -> ()
              n1371 = local write "单选_第45路"(w53) -> ()
              n1372 = local write "单选_第46路"(w53) -> ()
              n1373 = local write "单选_第47路"(w53) -> ()
              n1374 = local write "单选_第48路"(w53) -> ()
              n1375 = local write "单选_第49路"(w53) -> ()
              n1376 = local write "单选_第50路"(w53) -> ()
              n1377 = local write "单选_第51路"(w53) -> ()
              n1378 = local write "单选_第52路"(w53) -> ()
              n1379 = local write "单选_第53路"(w53) -> ()
              n1380 = local write "单选_第54路"(w53) -> ()
              n1381 = local write "单选_第55路"(w53) -> ()
              n1382 = local write "单选_第56路"(w53) -> ()
              n1383 = local write "单选_第57路"(w53) -> ()
              n1384 = local write "单选_第58路"(w53) -> ()
              n1385 = local write "单选_第59路"(w53) -> ()
              n1386 = local write "单选_第60路"(w53) -> ()
              n1387 = local write "单选_第61路"(w53) -> ()
              n1388 = local write "单选_第62路"(w53) -> ()
              n1389 = local write "单选_第63路"(w53) -> ()
              n1390 = local write "单选_第64路"(w53) -> ()
              n1391 = local write "单选_第71路"(w53) -> ()
              n1392 = local write "单选_第79路"(w53) -> ()
              n1393 = local write "单选_第65路"(w53) -> ()
              n1394 = local write "单选_第66路"(w53) -> ()
              n1395 = local write "单选_第67路"(w53) -> ()
              n1396 = local write "单选_第68路"(w53) -> ()
              n1397 = local write "单选_第69路"(w53) -> ()
              n1398 = local write "单选_第70路"(w53) -> ()
              n1399 = local write "单选_第72路"(w53) -> ()
              n1400 = local write "单选_第73路"(w53) -> ()
              n1401 = local write "单选_第74路"(w53) -> ()
              n1402 = local write "单选_第75路"(w53) -> ()
              n1403 = local write "单选_第76路"(w53) -> ()
              n1404 = local write "单选_第77路"(w53) -> ()
              n1405 = local write "单选_第78路"(w53) -> ()
              n1406 = local write "单选_第80路"(w53) -> ()
            }
            frame 13 {
              w54 = TRUE
              w55 = FALSE ("单选_第41路")
              n1407 = local write "单选_第1路"(w54) -> ()
              n1408 = local write "单选_第2路"(w54) -> ()
              n1409 = local write "单选_第3路"(w54) -> ()
              n1410 = local write "单选_第4路"(w54) -> ()
              n1411 = local write "单选_第5路"(w54) -> ()
              n1412 = local write "单选_第6路"(w54) -> ()
              n1413 = local write "单选_第7路"(w54) -> ()
              n1414 = local write "单选_第8路"(w54) -> ()
              n1415 = local write "单选_第9路"(w54) -> ()
              n1416 = local write "单选_第10路"(w54) -> ()
              n1417 = local write "单选_第11路"(w54) -> ()
              n1418 = local write "单选_第12路"(w54) -> ()
              n1419 = local write "单选_第13路"(w54) -> ()
              n1420 = local write "单选_第14路"(w55) -> ()
              n1421 = local write "单选_第15路"(w55) -> ()
              n1422 = local write "单选_第16路"(w55) -> ()
              n1423 = local write "单选_第17路"(w55) -> ()
              n1424 = local write "单选_第18路"(w55) -> ()
              n1425 = local write "单选_第19路"(w55) -> ()
              n1426 = local write "单选_第20路"(w55) -> ()
              n1427 = local write "单选_第21路"(w55) -> ()
              n1428 = local write "单选_第22路"(w55) -> ()
              n1429 = local write "单选_第23路"(w55) -> ()
              n1430 = local write "单选_第24路"(w55) -> ()
              n1431 = local write "单选_第25路"(w55) -> ()
              n1432 = local write "单选_第26路"(w55) -> ()
              n1433 = local write "单选_第27路"(w55) -> ()
              n1434 = local write "单选_第28路"(w55) -> ()
              n1435 = local write "单选_第29路"(w55) -> ()
              n1436 = local write "单选_第30路"(w55) -> ()
              n1437 = local write "单选_第31路"(w55) -> ()
              n1438 = local write "单选_第32路"(w55) -> ()
              n1439 = local write "单选_第33路"(w55) -> ()
              n1440 = local write "单选_第34路"(w55) -> ()
              n1441 = local write "单选_第35路"(w55) -> ()
              n1442 = local write "单选_第36路"(w55) -> ()
              n1443 = local write "单选_第37路"(w55) -> ()
              n1444 = local write "单选_第38路"(w55) -> ()
              n1445 = local write "单选_第39路"(w55) -> ()
              n1446 = local write "单选_第40路"(w55) -> ()
              n1447 = local write "单选_第41路"(w55) -> ()
              n1448 = local write "单选_第42路"(w55) -> ()
              n1449 = local write "单选_第43路"(w55) -> ()
              n1450 = local write "单选_第44路"(w55) -> ()
              n1451 = local write "单选_第45路"(w55) -> ()
              n1452 = local write "单选_第46路"(w55) -> ()
              n1453 = local write "单选_第47路"(w55) -> ()
              n1454 = local write "单选_第48路"(w55) -> ()
              n1455 = local write "单选_第49路"(w55) -> ()
              n1456 = local write "单选_第50路"(w55) -> ()
              n1457 = local write "单选_第51路"(w55) -> ()
              n1458 = local write "单选_第52路"(w55) -> ()
              n1459 = local write "单选_第53路"(w55) -> ()
              n1460 = local write "单选_第54路"(w55) -> ()
              n1461 = local write "单选_第55路"(w55) -> ()
              n1462 = local write "单选_第56路"(w55) -> ()
              n1463 = local write "单选_第57路"(w55) -> ()
              n1464 = local write "单选_第58路"(w55) -> ()
              n1465 = local write "单选_第59路"(w55) -> ()
              n1466 = local write "单选_第60路"(w55) -> ()
              n1467 = local write "单选_第61路"(w55) -> ()
              n1468 = local write "单选_第62路"(w55) -> ()
              n1469 = local write "单选_第63路"(w55) -> ()
              n1470 = local write "单选_第64路"(w55) -> ()
              n1471 = local write "单选_第71路"(w55) -> ()
              n1472 = local write "单选_第79路"(w55) -> ()
              n1473 = local write "单选_第65路"(w55) -> ()
              n1474 = local write "单选_第66路"(w55) -> ()
              n1475 = local write "单选_第67路"(w55) -> ()
              n1476 = local write "单选_第68路"(w55) -> ()
              n1477 = local write "单选_第69路"(w55) -> ()
              n1478 = local write "单选_第70路"(w55) -> ()
              n1479 = local write "单选_第72路"(w55) -> ()
              n1480 = local write "单选_第73路"(w55) -> ()
              n1481 = local write "单选_第74路"(w55) -> ()
              n1482 = local write "单选_第75路"(w55) -> ()
              n1483 = local write "单选_第76路"(w55) -> ()
              n1484 = local write "单选_第77路"(w55) -> ()
              n1485 = local write "单选_第78路"(w55) -> ()
              n1486 = local write "单选_第80路"(w55) -> ()
            }
            frame 14 {
              w56 = TRUE
              w57 = FALSE ("单选_第41路")
              n1487 = local write "单选_第1路"(w56) -> ()
              n1488 = local write "单选_第2路"(w56) -> ()
              n1489 = local write "单选_第3路"(w56) -> ()
              n1490 = local write "单选_第4路"(w56) -> ()
              n1491 = local write "单选_第5路"(w56) -> ()
              n1492 = local write "单选_第6路"(w56) -> ()
              n1493 = local write "单选_第7路"(w56) -> ()
              n1494 = local write "单选_第8路"(w56) -> ()
              n1495 = local write "单选_第9路"(w56) -> ()
              n1496 = local write "单选_第10路"(w56) -> ()
              n1497 = local write "单选_第11路"(w56) -> ()
              n1498 = local write "单选_第12路"(w56) -> ()
              n1499 = local write "单选_第13路"(w56) -> ()
              n1500 = local write "单选_第14路"(w56) -> ()
              n1501 = local write "单选_第15路"(w57) -> ()
              n1502 = local write "单选_第16路"(w57) -> ()
              n1503 = local write "单选_第17路"(w57) -> ()
              n1504 = local write "单选_第18路"(w57) -> ()
              n1505 = local write "单选_第19路"(w57) -> ()
              n1506 = local write "单选_第20路"(w57) -> ()
              n1507 = local write "单选_第21路"(w57) -> ()
              n1508 = local write "单选_第22路"(w57) -> ()
              n1509 = local write "单选_第23路"(w57) -> ()
              n1510 = local write "单选_第24路"(w57) -> ()
              n1511 = local write "单选_第25路"(w57) -> ()
              n1512 = local write "单选_第26路"(w57) -> ()
              n1513 = local write "单选_第27路"(w57) -> ()
              n1514 = local write "单选_第28路"(w57) -> ()
              n1515 = local write "单选_第29路"(w57) -> ()
              n1516 = local write "单选_第30路"(w57) -> ()
              n1517 = local write "单选_第31路"(w57) -> ()
              n1518 = local write "单选_第32路"(w57) -> ()
              n1519 = local write "单选_第33路"(w57) -> ()
              n1520 = local write "单选_第34路"(w57) -> ()
              n1521 = local write "单选_第35路"(w57) -> ()
              n1522 = local write "单选_第36路"(w57) -> ()
              n1523 = local write "单选_第37路"(w57) -> ()
              n1524 = local write "单选_第38路"(w57) -> ()
              n1525 = local write "单选_第39路"(w57) -> ()
              n1526 = local write "单选_第40路"(w57) -> ()
              n1527 = local write "单选_第41路"(w57) -> ()
              n1528 = local write "单选_第42路"(w57) -> ()
              n1529 = local write "单选_第43路"(w57) -> ()
              n1530 = local write "单选_第44路"(w57) -> ()
              n1531 = local write "单选_第45路"(w57) -> ()
              n1532 = local write "单选_第46路"(w57) -> ()
              n1533 = local write "单选_第47路"(w57) -> ()
              n1534 = local write "单选_第48路"(w57) -> ()
              n1535 = local write "单选_第49路"(w57) -> ()
              n1536 = local write "单选_第50路"(w57) -> ()
